vi "LogManyChannels.vi"() -> ()   [LabVIEW 2021]
uses:
  <vilib>/xnet/xnet.llb/XNET Create Session (Signal Input Waveform).vi
  <vilib>/xnet/xnet.llb/XNET Read (Signal Waveform) .vi
  <resource>/objmgr/xnet.rc
panel:
  out "error out":errorcluster
  out "Parsed Log file name":string
  in  "Log file name":string="LogFile_{Year}-{Month}-{Day}-{Hour}-{Minute}-{Second}.tdms"
  in  "Log file folder":path=path "C:/Users/NI/Desktop/Data"
  in  "Sample Rate (Hz)":dbl=100.0 format="%#_13g"
  in  "CAN Interface":refnum<k21>="CAN1"
  in  "XNET Cluster":refnum<k21>="ManyXnetChannels"
  out "#Signals":i32
  in  "stop":bool
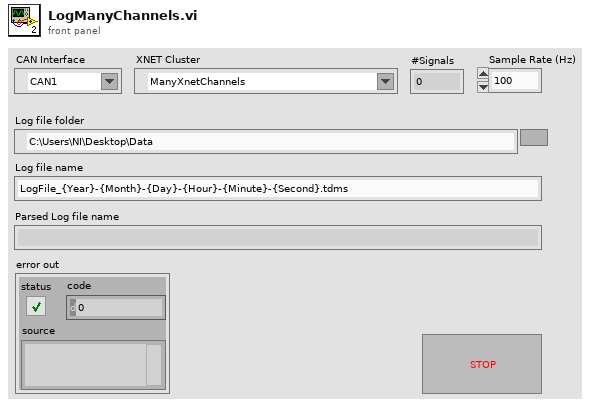
[diagram p1: front panel]
types:
  T1 = enum16{"open", "open or create", "create or replace", "create", "open (read-only)"}
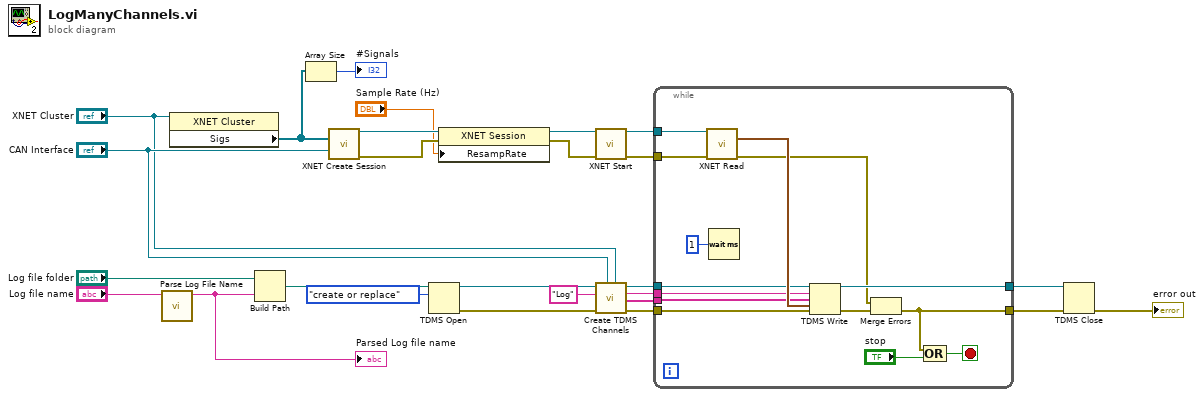
[diagram p0: block diagram]
diagram:
  n1 = call "Parse Log File Name.vi"("Log file name"="Log file name") -> ("Parsed Log file name"=w6:string)  [unwired: 10 in]
  "Parsed Log file name" <- w6
  n2 = property class="XNET Cluster"(reference="XNET Cluster") -> ("Sigs"=w17:refnum<k21>[])  [unwired: 1 in, 2 out]
  n3 = Build Path(base path="Log file folder", name or relative path=w6) -> (appended path=w11:path)
  n4 = Array Size(array=w17) -> (size(s)=→"#Signals":i32)
  n5 = call-poly <vilib>:"XNET Create Session.vi"("signal list"=w17, "interface"="CAN Interface") -> ("session out"=w26:refnum<k21>, "error out"=w25:errorcluster)  [unwired: 12 in]
  n6 = TDMS Open(10:T1."create or replace" ("operation (0:open)"), 11:w11) -> (0:w14:errorcluster, 3:w16:refnum<k34>)  [unwired: 5 in]
  n7 = property class="XNET Session"(reference=w26, error in=w25, "ResampRate"="Sample Rate (Hz)") -> (reference out=w22:refnum<k21>, error out=w21:errorcluster)
  n8 = call <vilib>:"XNET Start.vi"("session in"=w22, "error in (no error)"=w21) -> ("session out"=w19:refnum<k21>, "error out"=w20:errorcluster)  [unwired: 12 in]
  n9 = call "Create TDMS Channels.vi"("XNET Cluster"="XNET Cluster", "CAN Interface"="CAN Interface", "error in (no error)"=w14, "group name in"="Log", "TDMS ref in"=w16) -> ("error out"=w13:errorcluster, "Signal Names"=w7:string[], "group name out"=w8:string, "TDMS ref out"=w15:refnum<k34>)  [unwired: 3 in]
  n10 = while {
    tunnel: w19 -> [w40]
    tunnel: w20 -> [w39]
    tunnel: [w34] -> w18
    tunnel: w7 -> [w32]
    tunnel: w15 -> [w31]
    tunnel: w13 -> [w30]
    tunnel: w8 -> [w29]
    tunnel: [w27] -> w4
    stop <- w37 stop-if-true
    n11 = call-poly <vilib>:"XNET Read.vi"("session in"=w40, "error in (no error)"=w39) -> ("data"=w35:waveform(dbl)[], "error out"=w28:errorcluster)  [unwired: 11 in, 1 out]
    n12 = Wait (ms)(milliseconds to wait=u32 1) -> ()  [unwired: 1 out]
    n13 = TDMS Write(0:w31, 5:w29, 7:w32, 9:w35, 11:w30) -> (4:w34:refnum<k34>, 15:w33:errorcluster)  [unwired: 1 in, 2 out]
    n14 = Merge Errors(w28, w33) -> (w27:errorcluster)
    n15 = Compound Arithmetic op=OR(w27, "stop") -> (w37:bool)
  }
  n16 = TDMS Close(8:w4, 11:w18) -> (0:→"error out":errorcluster)  [unwired: 1 out]
